vi "Start New Set.vi"(8 "error in (no error)":errorcluster, 10 "Parameter":refnum<class "AbstractData.lvclass">, 11 "StorageService in":refnum<class "StorageService.lvclass">) -> (0 "error out":errorcluster, 3 "StorageService out":refnum<class "StorageService.lvclass">)   [LabVIEW 2014, in "StorageService.lvclass"]
uses:
  StorageService.lvclass
  Model/Data/AbstractData/AbstractData.lvclass
  StorageService.lvclass/StorageService.ctl
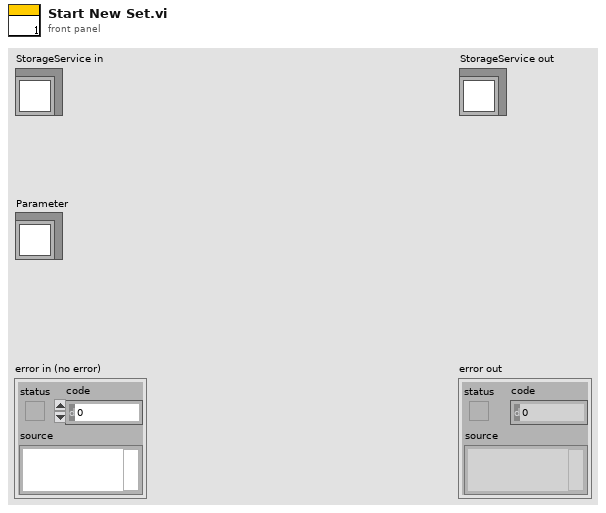
[diagram p1: front panel]
types:
  T1 = typedef "StorageService.lvclass/RegisteredObject.ctl" = cluster{"Name":string, "Is Acquired":bool, "Queue":refnum<queue>, "Message To Send":cluster{"Enqueuer":refnum<class "Message Enqueuer.lvclass">, "Message":refnum<class "ReplayData Msg.lvclass">}, "Save Parameters":variant}
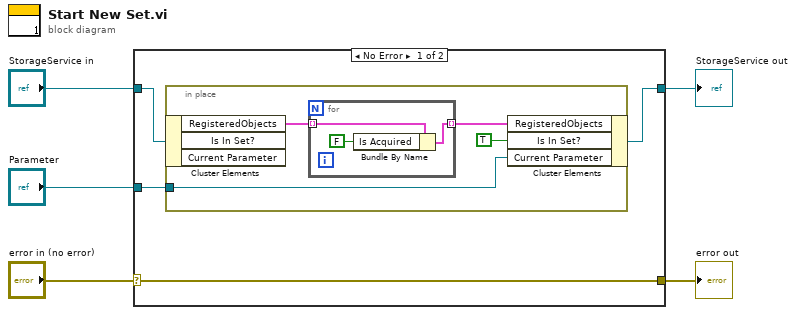
[diagram p0: block diagram]
diagram:
  n1 = case shown="No Error" "error in (no error)" {
    selector: "error in (no error)" -> [w9 w18]
    tunnel: [w9 w18] -> w4
    tunnel: [w6 w17] -> w2
    tunnel: "StorageService in" -> [w7 w17]
    tunnel: "Parameter" -> [w8 _]
    frame No Error {
      n2 = in-place {
        in-place-border: w8 -> [w10]
        n3 = in-place-cluster #1(w7) -> ("RegisteredObjects"=w13:T1[])  [unwired: 2 out]
        n4 = for {
          tunnel: w13 -> [w16] mode=indexing
          tunnel: [w14] -> w12 mode=indexing
          n5 = Bundle By Name(cluster=w16, "Is Acquired"=FALSE) -> (w14:T1)
        }
        n6 = in-place-cluster #1("RegisteredObjects"=w12, "Is In Set?"=TRUE, "Current Parameter"=w10) -> (w6:refnum<class "StorageService.lvclass">)
      }
    }
    frame Error {
    }
  }
  "error out" <- w4
  "StorageService out" <- w2
